vi "_word.table.Content.vi"(7 "word.application":refnum<k7>, 8 "error in (no error)":errorcluster, 11 "table in":refnum<k7>) -> (0 "error out":errorcluster, 2 "table row contents":string[][](array[string]), 3 "table out":refnum<k7>)   [LabVIEW 2018, in "WordReportGeneration.lvlib"]
uses:
  WordReportGeneration.lvlib
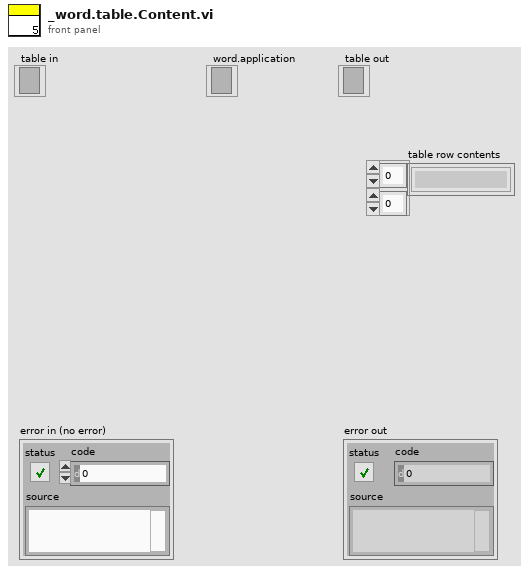
[diagram p1: front panel]
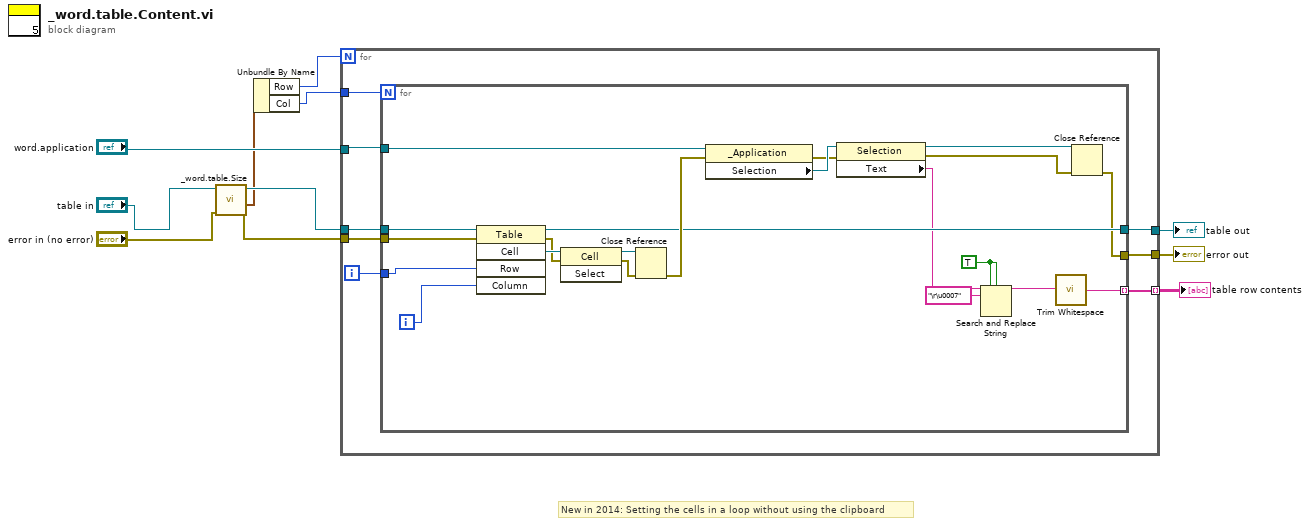
[diagram p0: block diagram]
diagram:
  # "New in 2014: Setting the cells in a loop without using the clipboard"
  n1 = call "_word.table.Size.vi"("error in (no error)"="error in (no error)", "table Refnum in"="table in") -> ("error out"=w5:errorcluster, "Cluster"=w3:cluster{"Row":i32, "Col":i32}, "table Refnum out"=w7:refnum<k7>)  [unwired: 7 in]
  n2 = Unbundle By Name(w3) -> ("Row"=w2:i32, "Col"=w1:i32)
  n3 = for {
    N: w2 -> [_]
    tunnel: [w19] -> w10
    tunnel: [w18] -> w11
    tunnel: w5 -> [w16]
    tunnel: "word.application" -> [w15]
    tunnel: w7 -> [w14]
    tunnel: [w13] -> w4 mode=indexing
    tunnel: w1 -> [w12]
    i -> [w17]
    n4 = for {
      N: w12 -> [_]
      tunnel: [w35] -> w19
      tunnel: [w29] -> w18
      tunnel: w17 -> [w26]
      tunnel: w16 -> [w34]
      tunnel: w15 -> [w33]
      tunnel: w14 -> [w32]
      tunnel: [w24] -> w13 mode=indexing
      i -> [w25]
      w21 = TRUE ("ignore case? (F)")
      n5 = invoke class="Table" method="Cell"(reference=w32, error in=w34, "Row"=w26, "Column"=w25) -> (reference out=w35:refnum<k7>, error out=w39:errorcluster, "Cell"=w40:refnum<k7>)  [unwired: 1 in, 2 out]
      n6 = invoke class="Cell" method="Select"(reference=w40, error in=w39) -> (reference out=w36:refnum<k7>, error out=w38:errorcluster)  [unwired: 1 in, 1 out]
      n7 = Close Reference(reference=w36, error in (no error)=w38) -> (error out=w37:errorcluster)
      n8 = property class="_Application"(reference=w33, error in=w37) -> (error out=w27:errorcluster, "Selection"=w28:refnum<k7>)  [unwired: 1 out]
      n9 = property class="Selection"(reference=w28, error in=w27) -> (reference out=w30:refnum<k7>, error out=w31:errorcluster, "Text"=w22:string)
      n10 = Search and Replace String(replace all?=w21, case sensitive?=w21, input string=w22, search string="\r\u0007") -> (result string=w23:string)  [unwired: 4 in, 3 out]
      n11 = call <vilib>:"Trim Whitespace.vi"("string"=w23) -> ("trimmed string"=w24:string)  [unwired: 1 in]
      n12 = Close Reference(reference=w30, error in (no error)=w31) -> (error out=w29:errorcluster)
    }
  }
  "error out" <- w11
  "table out" <- w10
  "table row contents" <- w4
